vi "Get SubRoutines.vi"(11 "Path":path) -> (3 "SubRoutine Profile":i32[][](array[numeric]))   [LabVIEW 2013]
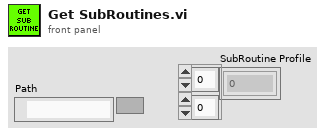
[diagram p1: front panel]
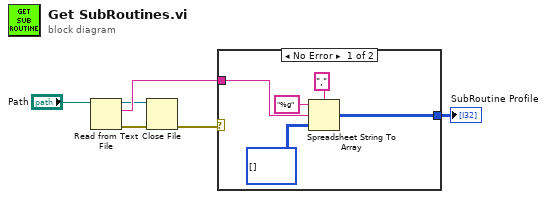
[diagram p0: block diagram]
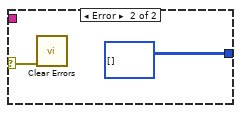
[diagram p2: hidden frame]
diagram:
  n1 = Read from Text File(file (use dialog)="Path") -> (refnum out=w5:refnum<file>, text=w6:string, error out=w4:errorcluster)  [unwired: 3 in, 1 out]
  n2 = Close File(refnum=w5, error in=w4) -> (error out=w2:errorcluster)  [unwired: 1 out]
  n3 = case shown="No Error" w2 {
    selector: w2 -> [_ w13]
    tunnel: w6 -> [w9 _]
    tunnel: [w7 i32[][] []] -> w1
    frame No Error {
      n4 = Spreadsheet String To Array(delimiter (Tab)=",", format string="%g", spreadsheet string=w9, array type (2D Dbl)=i32[][] []) -> (array=w7:i32[][])
    }
    frame Error {
      n5 = call <vilib>:"Clear Errors.vi"("error in (no error)"=w13) -> ()  [unwired: 6 in, 1 out]
    }
  }
  "SubRoutine Profile" <- w1
